vi "RT Main.vi"() -> ()   [LabVIEW 2013]
uses:
  <vilib>/NI/Current Value Table/Type Defs/Single Tag.ctl
  <vilib>/NI/Current Value Table/Type Defs/Data Types.ctl
  <userlib>/CIE/_TypeDefs/CIE Configuration.ctl
  <vilib>/NI/Current Value Table/Compatibility/_SubVIs/TypeDefs/cvt_Tag Configuration.ctl
  <vilib>/NI/Current Value Table/Compatibility/_SubVIs/TypeDefs/cvt_Data Types.ctl
  <vilib>/NI/Current Value Table/Type Defs/File Format.ctl
  <vilib>/NI/Current Value Table/Type Defs/Tag Grouping set.ctl
  <vilib>/NI/CCC/CIE Tag Configuration.ctl
  <vilib>/NI/Current Value Table/Write.vi
  <vilib>/NI/Current Value Table/DataTypes/Boolean_Write.vi
  <vilib>/NI/Current Value Table/Type to Enum.vi
  <vilib>/NI/Current Value Table/DataTypes/Boolean_Type To Enum.vi
  <vilib>/Utility/file.llb/Read From Spreadsheet File (string).vi
  <vilib>/NI/Current Value Table/FGVs/CVT Globals.vi
  <vilib>/NI/Current Value Table/FGVs/Tag Memory.vi
  <vilib>/NI/Current Value Table/Memory Block.vi
  <vilib>/NI/Current Value Table/DataTypes/Boolean_Memory Block.vi
  <vilib>/NI/Current Value Table/Current Value Table.lvlib
  <vilib>/NI/CCC/NI_CCC.lvlib
  <vilib>/NI/AMC/AMC.lvlib
panel:
  out "output cluster 2":T1
  out "output cluster":T1
  out "CVT Tags":T4[](array[typedef])
  out "Invalid  CVT Tags":T4[](array[typedef])
  in  "Stop":bool
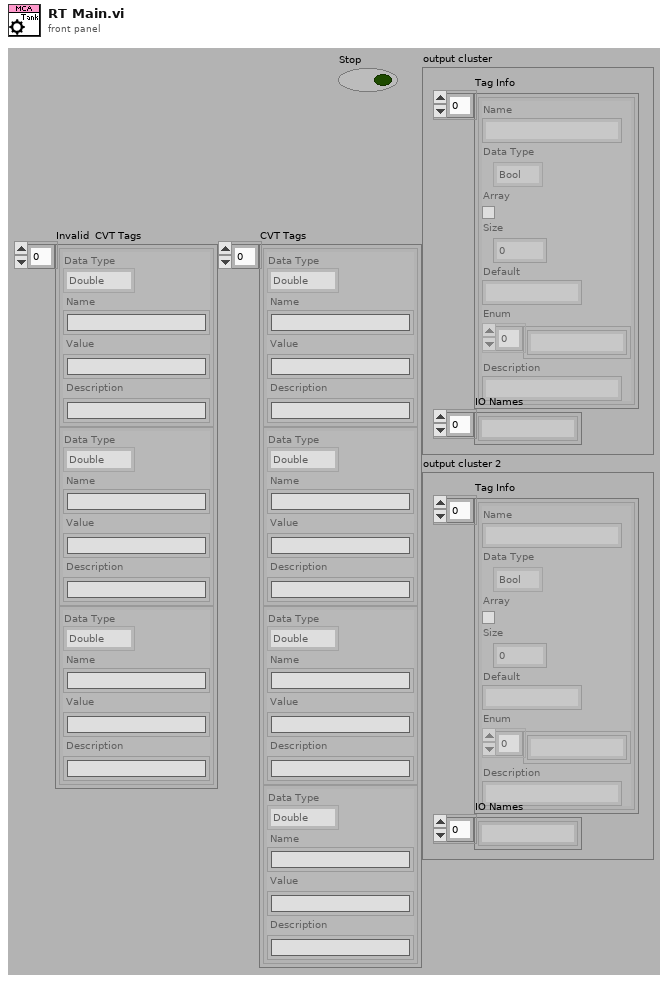
[diagram p1: front panel]
types:
  T1 = typedef "CIE Configuration.ctl" = cluster{"Tag Info":T2[], "IO Names":string[]}
  T2 = typedef "cvt_Tag Configuration.ctl" = cluster{"Name":string, "Data Type":T3, "Array":bool, "Size":u32, "Default":string, "Enum":string[], "Description":string}
  T3 = typedef "cvt_Data Types.ctl" = enum16{"Bool", "U8", "I32", "Double", "String", "Enum"}
  T4 = typedef "Current Value Table.lvlib/Single Tag.ctl" = cluster{"Data Type":T5, "Name":string, "Value":string, "Description":string}
  T5 = typedef "Current Value Table.lvlib/Data Types.ctl" = enum16{"Double", "Single", "I64", "I32", "I16", "I8", "U64", "U32", "U16", "U8", "String", "Boolean", "Array of U8", "Array of U16", "Array of U32", "Array of U64", "Array of I64", "Array of I32", "Array of I16", "Array of I8", "Array of Double", "Array of Single", "Array of Boolean", "Array of String"}
  T6 = typedef "Current Value Table.lvlib/File Format.ctl" = cluster{"Tags":T4[], "Group Listings":T7[]}
  T7 = typedef "Current Value Table.lvlib/Tag Grouping set.ctl" = cluster{"Group":string, "Tag Names":string[]}
  T8 = typedef "CIE Tag Configuration.ctl" = cluster{"Name":string, "Data Type":T3, "Array":bool, "Size":u32, "Default":string, "Enum":string[], "Description":string}
  T9 = typedef "CIE Tags.ctl" = cluster{"DBL Tags":T10[], "BOOL Tags":T11[], "I32 Tags":T12[], "ENUM Tags":T13[], "STR Tags":T14[]}
  T10 = typedef "DBL CIE Tag.ctl" = cluster{"Tag Index":i32, "Output?":bool, "SV Ref":refnum<k21>, "CVT Tag":string}
  T11 = typedef "BOOL CIE Tag.ctl" = cluster{"Tag Index":i32, "Output?":bool, "SV Ref":refnum<k21>, "CVT Tag":string}
  T12 = typedef "I32 CIE Tag.ctl" = cluster{"Tag Index":i32, "Output?":bool, "SV Ref":refnum<k21>, "CVT Tag":string}
  T13 = typedef "Enum CIE Tag.ctl" = cluster{"Tag Index":i32, "Output?":bool, "SV Ref":refnum<k21>, "CVT Tag":string}
  T14 = typedef "STR CIE Tag.ctl" = cluster{"Tag Index":i32, "Output?":bool, "SV Ref":refnum<k21>, "CVT Tag":string}
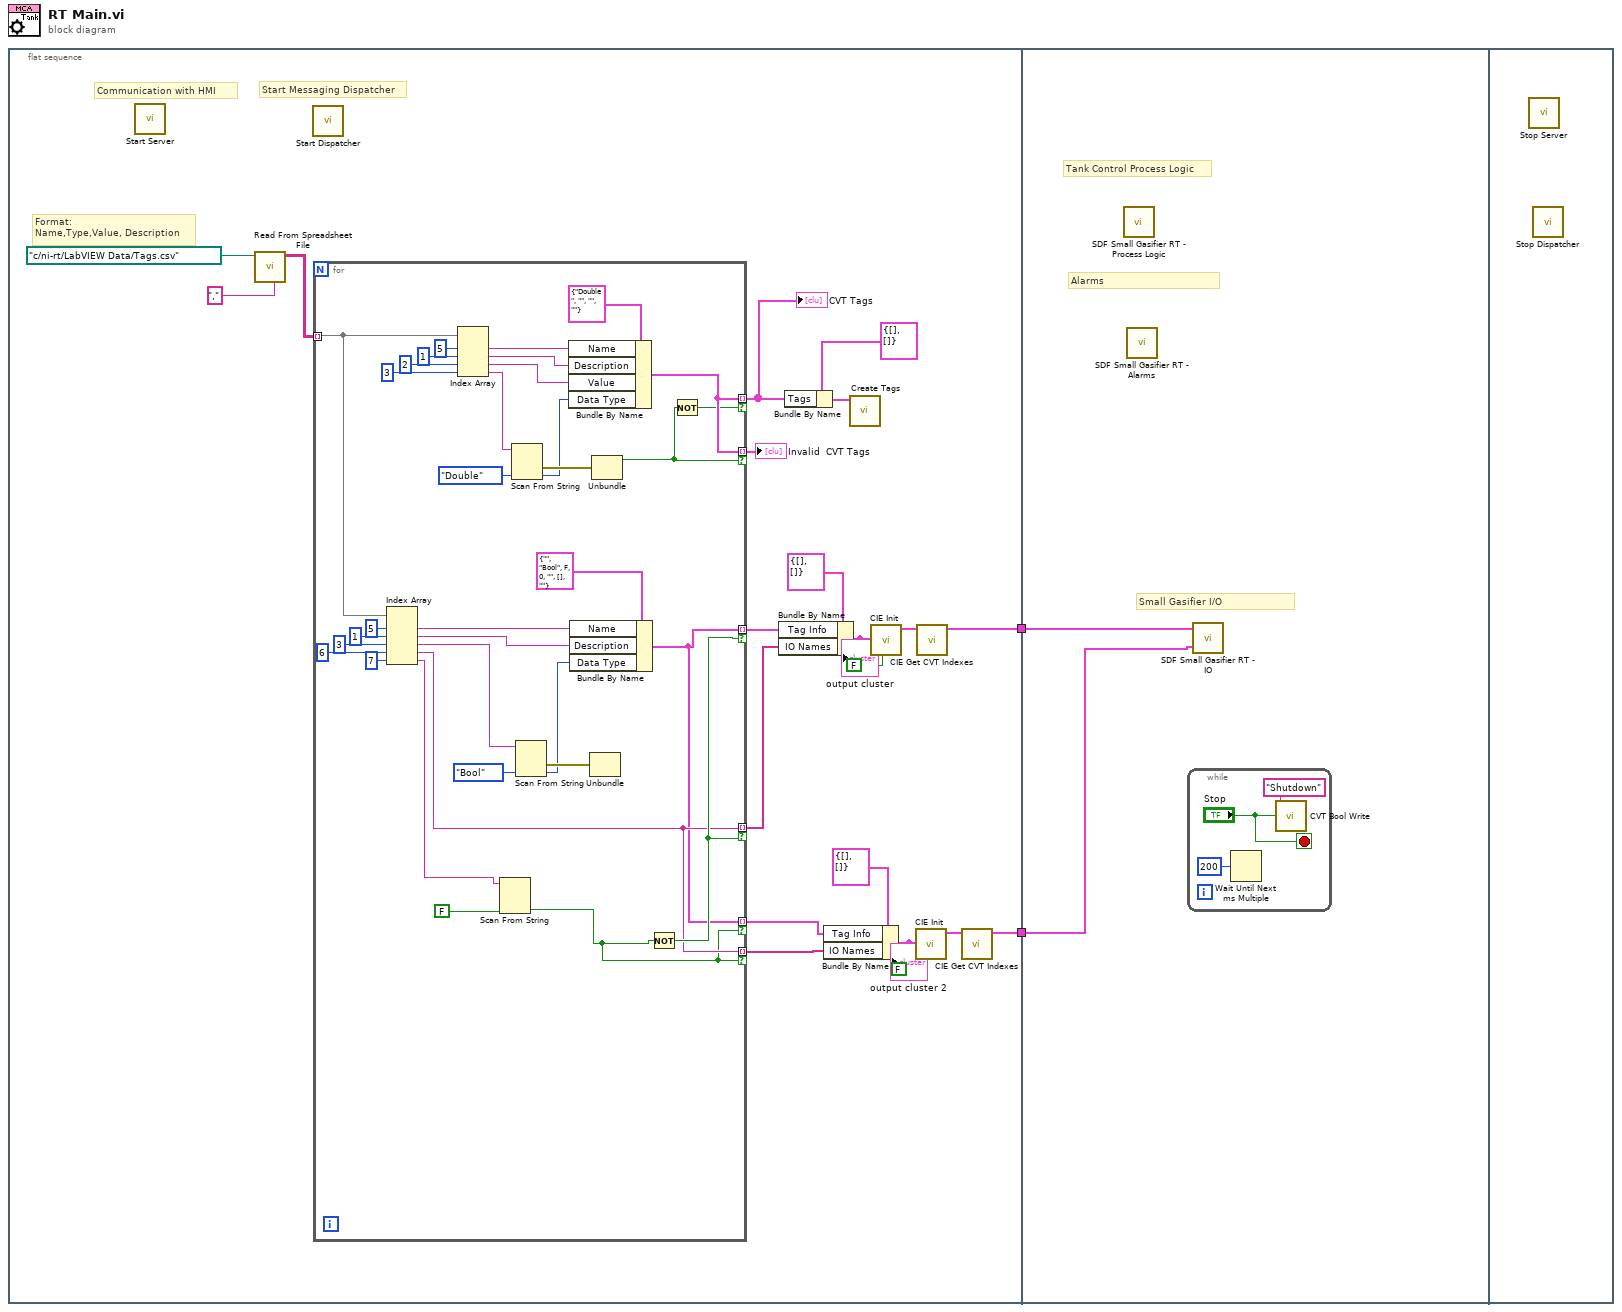
[diagram p0: block diagram]
diagram:
  n1 = flat-sequence {
    tunnel: [w11] -> w2
    tunnel: [w4] -> w1
    tunnel: w2 -> [w59]
    tunnel: w1 -> [w58]
    frame #0 {
      # "Format:\nName,Type,Value, Description"
      # "Start Messaging Dispatcher"
      # "Communication with HMI"
      n2 = call <vilib>:"Start Server.vi"() -> ()  [unwired: 11 in, 1 out]
      n3 = call-poly <vilib>:"Read From Spreadsheet File.vi"("delimiter (\\t)"="," ("delimiter (\\t)"), "file path (dialog if empty)"=path "c:/ni-rt/LabVIEW Data/Tags.csv") -> ("all rows"=w17:string[][])  [unwired: 5 in, 4 out]
      n4 = call <vilib>:"Start Dispatcher.vi"() -> ()  [unwired: 13 in, 3 out]
      n5 = for {
        tunnel: w17 -> [w41] mode=indexing
        tunnel: [w54] -> w20 mode=indexing if=w52
        tunnel: [w54] -> w22 mode=indexing if=w53
        tunnel: [w25] -> w15 mode=indexing if=w27
        tunnel: [w26] -> w14 mode=indexing if=w27
        tunnel: [w26] -> w5 mode=indexing if=w24
        tunnel: [w25] -> w3 mode=indexing if=w24
        n6 = Index Array(array=w41, index #1=5 ("index"), index #2=1 ("index"), index #3=3 ("index"), index #4=6 ("index"), index #5=7 ("index")) -> (element #1=w40:string, element #2=w38:string, element #3=w37:string, element #4=w26:string, element #5=w28:string)
        n7 = Index Array(array=w41, index #1=5 ("index"), index #2=1 ("index"), index #3=2 ("index"), index #4=3 ("index")) -> (element #1=w56:string, element #2=w46:string, element #3=w45:string, element #4=w44:string)
        n8 = Scan From String(input string=w28, default 1=FALSE ("Boolean")) -> (output 1=w24:bool)  [unwired: 3 in, 3 out]
        n9 = Scan From String(input string=w44, default 1=Data_Types."Double" ("Data Type")) -> (error out=w55:errorcluster, output 1=w43:T5)  [unwired: 3 in, 2 out]
        n10 = Scan From String(input string=w37, default 1=cvt_Data_Types."Bool" ("Data Type")) -> (error out=w39:errorcluster, output 1=w35:T3)  [unwired: 3 in, 2 out]
        n11 = Bundle By Name(cluster=T4 {"Data Type"=enum."Double", "Name"="", "Value"="", "Description"=""} ("Tag"), "Name"=w56, "Description"=w46, "Value"=w45, "Data Type"=w43) -> (w54:T4)
        n12 = Bundle By Name(cluster=T8 {"Name"="", "Data Type"=enum."Bool", "Array"=FALSE, "Size"=0, "Default"="", "Enum"=[], "Description"=""} ("Tag Info"), "Name"=w40, "Description"=w38, "Data Type"=w35) -> (w25:T8)
        n13 = Unbundle(w39) -> ()  [unwired: 3 out]
        n14 = Unbundle(w55) -> ("status"=w52:bool)  [unwired: 2 out]
        n15 = Not(x=w24) -> (.not. x?=w27:bool)
        n16 = Not(x=w52) -> (.not. x?=w53:bool)
      }
      "Invalid  CVT Tags" <- w20
      "CVT Tags" <- w22
      n17 = Bundle By Name(cluster=T1 {"Tag Info"=[], "IO Names"=[]} ("Configuration"), "Tag Info"=w15, "IO Names"=w14) -> (w13:T1)
      "output cluster" <- w13
      n18 = Bundle By Name(cluster=T6 {"Tags"=[], "Group Listings"=[]} ("CVT Tags to Create"), "Tags"=w22) -> (w19:T6)
      n19 = Bundle By Name(cluster=T1 {"Tag Info"=[], "IO Names"=[]} ("Configuration"), "Tag Info"=w3, "IO Names"=w5) -> (w8:T1)
      "output cluster 2" <- w8
      n20 = call <vilib>:"Create Tags.vi"("CVT Tags to Create"=w19) -> ()  [unwired: 10 in, 1 out]
      n21 = call <userlib>:"CIE Init.vi"("Use Unconfigured Channels?"=FALSE, "Configuration"=w13) -> ("CIE Tags"=w12:T9)  [unwired: 6 in, 3 out]
      n22 = call <userlib>:"CIE Init.vi"("Use Unconfigured Channels?"=FALSE, "Configuration"=w8) -> ("CIE Tags"=w7:T9)  [unwired: 6 in, 3 out]
      n23 = call <userlib>:"CIE Get CVT Indexes.vi"("CIE Tags In"=w12) -> ("CIE Tags Out"=w11:T9)  [unwired: 9 in, 1 out]
      n24 = call <userlib>:"CIE Get CVT Indexes.vi"("CIE Tags In"=w7) -> ("CIE Tags Out"=w4:T9)  [unwired: 9 in, 1 out]
    }
    frame #1 {
      # "Alarms"
      # "Tank Control Process Logic"
      # "Small Gasifier I/O"
      n25 = call "SDF Small Gasifier RT - Process Logic.vi"() -> ()  [unwired: 12 in]
      n26 = call "SDF Small Gasifier RT - Alarms.vi"() -> ()  [unwired: 1 in]
      n27 = while {
        stop <- "Stop" stop-if-true
        n28 = Wait Until Next ms Multiple(millisecond multiple=u32 200) -> ()  [unwired: 1 out]
        n29 = call <vilib>:"CVT Bool Write.vi"("Value"="Stop", "Tag Name"="Shutdown") -> ()  [unwired: 3 in, 1 out]
      }
      n30 = call "SDF Small Gasifier RT - IO.vi"("CIE Tags 2"=w58, "CIE Tags"=w59) -> ()
    }
    frame #2 {
      n31 = call <vilib>:"Stop Server.vi"() -> ()  [unwired: 11 in, 1 out]
      n32 = call <vilib>:"Stop Dispatcher.vi"() -> ()  [unwired: 15 in, 1 out]
    }
  }
